vi "_r2dio_8in_8out_canopen_master.vi"() -> ()   [LabVIEW 2011]
uses:
  CANopen_VI/stop_can_master.vi
panel:
  out "ret transmit_can_pdo":i16
  out "datasize":u32
  out "Manufacturer software ver":string
  out "ret read_device_object_sdo 3":i16
  out "datasize":u32
  out "Manufacturer hardware ver":string
  out "ret read_device_object_sdo 2":i16
  out "datasize":u32
  out "Manufacturer dev name":string
  out "ret read_device_object_sdo 1":i16
  out "ret write_node_object_dictionary":i16
  in  "7":bool
  in  "6":bool
  in  "5":bool
  in  "4":bool
  in  "3":bool
  in  "2":bool
  in  "1":bool
  in  "0":bool
  out "ret write_pdo_mapping 6":i16
  out "ret write_pdo_mapping 5":i16
  out "ret write_pdo_mapping 4":i16
  out "ret add_node_object_dictionary 6200":i16
  out "7":bool
  out "6":bool
  out "5":bool
  out "4":bool
  out "3":bool
  out "2":bool
  out "1":bool
  out "0":bool
  out "7":bool
  out "6":bool
  out "5":bool
  out "4":bool
  out "3":bool
  out "2":bool
  out "1":bool
  out "0":bool
  out "uns8":u8
  out "upd":u8
  out "ret read_node_object_dictionary":i16
  in  "stop monitor":bool
  out "ret write_master_hbt":i16
  out "ret stop_can_master":i16
  out "ret write_pdo_mapping 3":i16
  out "ret write_pdo_mapping 2":i16
  out "ret write_pdo_mapping 1":i16
  out "ret add_node_object_dictionary 6000":i16
  out "ret write_device_object_sdo":i16
  in  "slave node":u8
  in  "baudrate":T1(ring)
  in  "net":u8
  # "Inputs"
  # "Outputs"
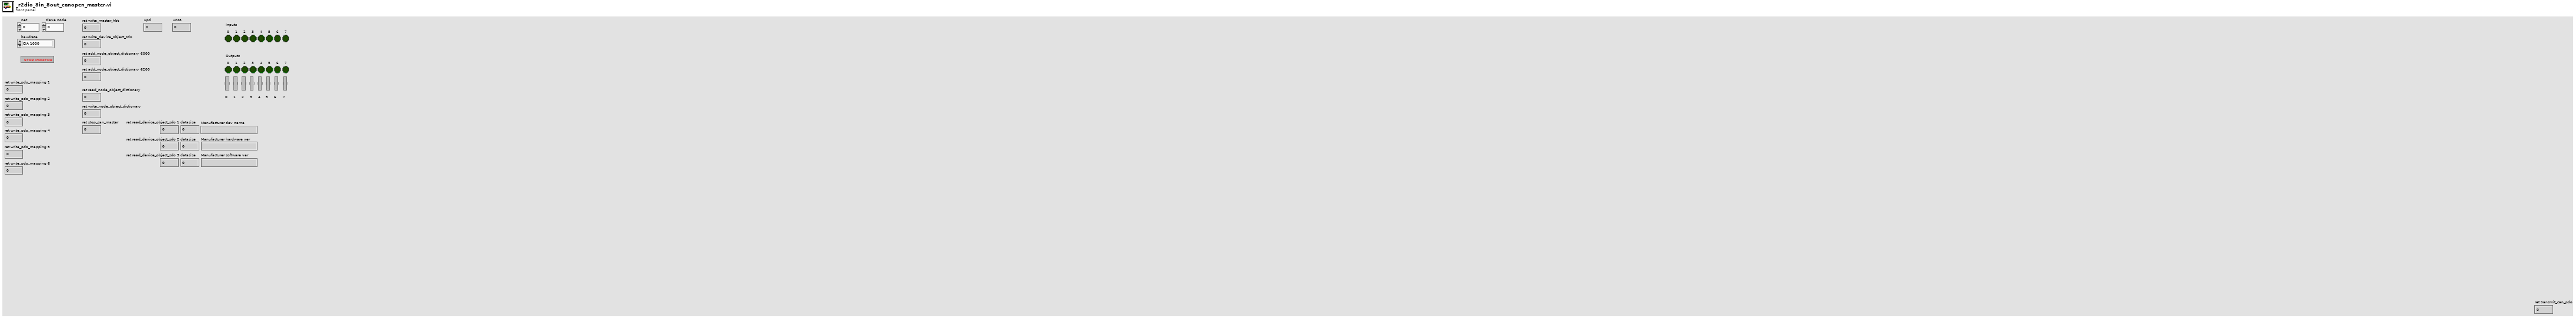
[diagram p1: front panel]
types:
  T1 = enum8{"CIA 1000", "CIA 800", "CIA 500", "CIA 250", "CIA 125", "CIA 100", "CIA 50", "CIA 20", "CIA 10", "CIA AUTO"}
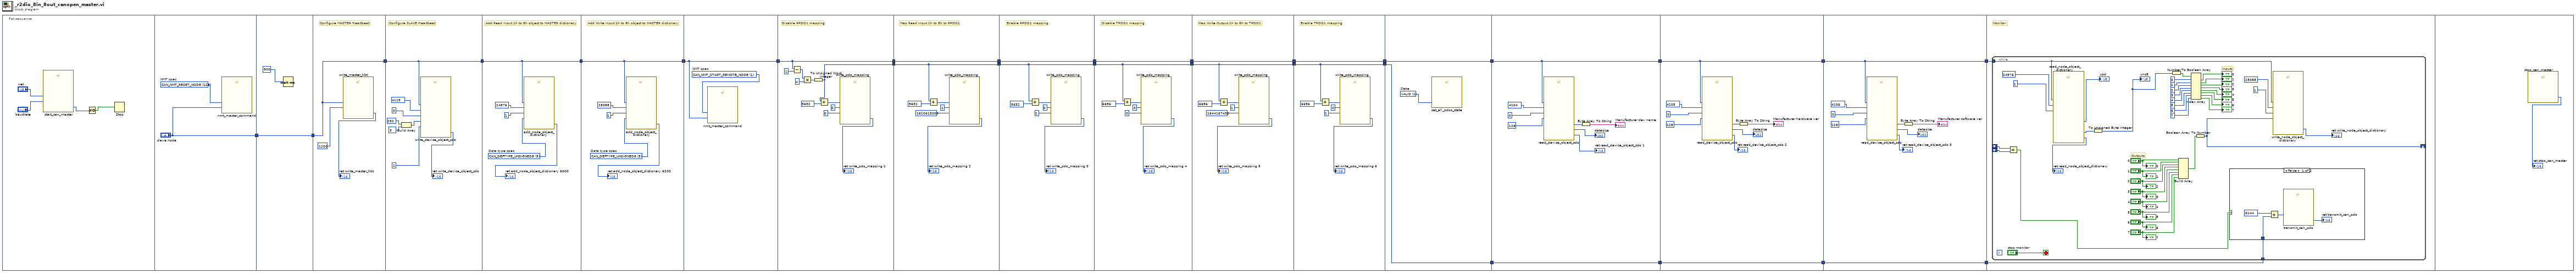
[diagram p0: block diagram]
diagram:
  n1 = flat-sequence {
    tunnel: ["slave node"] -> w25
    tunnel: w25 -> [w35]
    tunnel: [w35] -> w24
    tunnel: w24 -> [w37]
    tunnel: [w37] -> w27
    tunnel: w27 -> [w44]
    tunnel: [w44] -> w26
    tunnel: w26 -> [w47]
    tunnel: [w47] -> w20
    tunnel: w20 -> [w52]
    tunnel: [w52] -> w19
    tunnel: [w57] -> w21
    tunnel: w19 -> [w57]
    tunnel: [w62] -> w22
    tunnel: w21 -> [w62]
    tunnel: [w59] -> w10
    tunnel: [w73] -> w23
    tunnel: w22 -> [w73]
    tunnel: w10 -> [w70]
    tunnel: [w70] -> w9
    tunnel: [w80] -> w18
    tunnel: w23 -> [w80]
    tunnel: w9 -> [w77]
    tunnel: [w77] -> w8
    tunnel: w18 -> [w90]
    tunnel: [w90] -> w17
    tunnel: w8 -> [w84]
    tunnel: [w84] -> w7
    tunnel: w17 -> [w97]
    tunnel: [w97] -> w16
    tunnel: w7 -> [w91]
    tunnel: [w91] -> w6
    tunnel: w16 -> [w104]
    tunnel: [w104] -> w15
    tunnel: w6 -> [w98]
    tunnel: [w98] -> w1
    tunnel: [w106] -> w14
    tunnel: w15 -> [w106]
    tunnel: [w105] -> w2
    tunnel: w1 -> [w105]
    tunnel: w14 -> [w116]
    tunnel: [w116] -> w13
    tunnel: [w108] -> w3
    tunnel: w2 -> [w108]
    tunnel: w13 -> [w118]
    tunnel: [w118] -> w12
    tunnel: [w117] -> w4
    tunnel: w3 -> [w117]
    tunnel: w12 -> [w127]
    tunnel: [w127] -> w11
    tunnel: [w126] -> w5
    tunnel: w4 -> [w126]
    tunnel: w11 -> [w136]
    tunnel: w5 -> [w135]
    frame #0 {
      n2 = call "start_can_master.vi"("br"="baudrate", "net"="net") -> ("return"=w31:i16)  [unwired: 9 in]
      n3 = Not Equal To 0?(x=w31) -> (x != 0?=w30:bool)
      n4 = Stop(stop? (T)=w30) -> ()
    }
    frame #1 {
      w33 = u8 129 items=["CAN_NMT_CS_DUMMY"=0, "CAN_NMT_START_REMOTE_NODE"=1, "CAN_NMT_STOP_REMOTE_NODE"=2, "CAN_NMT_ENTER_PRE_OPERATIONAL"=128, "CAN_NMT_RESET_NODE"=129, "CAN_NMT_RESET_COMMUNICATION"=130]  # NMT spec
      n5 = call "nmt_master_command.vi"("node"="slave node", "cs"=w33) -> ()  [unwired: 10 in]
    }
    frame #2 {
      n6 = Wait (ms)(milliseconds to wait=u32 500) -> ()  [unwired: 1 out]
    }
    frame #3 {
      # "Configure MASTER Heartbeat"
      n7 = call "write_master_hbt.vi"("hbt"=u16 1200, "node"=w37) -> ("return"=→"ret write_master_hbt":i16)  [unwired: 9 in]
    }
    frame #4 {
      # "Configure SLAVE Heartbeat"
      n8 = Build Array(u8 232, u8 3) -> (w40:u8[])
      n9 = call "write_device_object_sdo.vi"("node"=w44, "index"=u16 4119, "subind"=u8 0, "data"=w40, "datasize"=u32 2) -> ("return"=→"ret write_device_object_sdo":i16)  [unwired: 10 in]
    }
    frame #5 {
      w49 = u16 5 items=["CAN_DEFTYPE_BOOLEAN"=1, "CAN_DEFTYPE_INTEGER8"=2, "CAN_DEFTYPE_INTEGER16"=3, "CAN_DEFTYPE_INTEGER32"=4, "CAN_DEFTYPE_UNSIGNED8"=5, "CAN_DEFTYPE_UNSIGNED16"=6, "CAN_DEFTYPE_UNSIGNED32"=7, "CAN_DEFTYPE_REAL32"=8, "CAN_DEFTYPE_VISIBLE_STRING"=9, "CAN_DEFTYPE_OCTET_STRING"=10, "CAN_DEFTYPE_UNICODE_STRING"=11, "CAN_DEFTYPE_TIME_OF_DAY"=12, "CAN_DEFTYPE_TIME_DIFFERENCE"=13, "CAN_DEFTYPE_DOMAIN"=15, "CAN_DEFTYPE_INTEGER24"=16, "CAN_DEFTYPE_REAL64"=17, "CAN_DEFTYPE_INTEGER40"=18, "CAN_DEFTYPE_INTEGER48"=19, "CAN_DEFTYPE_INTEGER56"=20, "CAN_DEFTYPE_INTEGER64"=21, "CAN_DEFTYPE_UNSIGNED24"=22, "CAN_DEFTYPE_UNSIGNED40"=24, "CAN_DEFTYPE_UNSIGNED48"=25, "CAN_DEFTYPE_UNSIGNED56"=26, "CAN_DEFTYPE_UNSIGNED64"=27]  # Data type spec
      # "Add Read Input 1h to 8h object to MASTER dictionary"
      n10 = call "add_node_object_dictionary.vi"("type"=w49, "subind"=u8 1, "index"=u16 24576, "node"=w47) -> ("return"=→"ret add_node_object_dictionary 6000":i16)  [unwired: 7 in]
    }
    frame #6 {
      w54 = u16 5 items=["CAN_DEFTYPE_BOOLEAN"=1, "CAN_DEFTYPE_INTEGER8"=2, "CAN_DEFTYPE_INTEGER16"=3, "CAN_DEFTYPE_INTEGER32"=4, "CAN_DEFTYPE_UNSIGNED8"=5, "CAN_DEFTYPE_UNSIGNED16"=6, "CAN_DEFTYPE_UNSIGNED32"=7, "CAN_DEFTYPE_REAL32"=8, "CAN_DEFTYPE_VISIBLE_STRING"=9, "CAN_DEFTYPE_OCTET_STRING"=10, "CAN_DEFTYPE_UNICODE_STRING"=11, "CAN_DEFTYPE_TIME_OF_DAY"=12, "CAN_DEFTYPE_TIME_DIFFERENCE"=13, "CAN_DEFTYPE_DOMAIN"=15, "CAN_DEFTYPE_INTEGER24"=16, "CAN_DEFTYPE_REAL64"=17, "CAN_DEFTYPE_INTEGER40"=18, "CAN_DEFTYPE_INTEGER48"=19, "CAN_DEFTYPE_INTEGER56"=20, "CAN_DEFTYPE_INTEGER64"=21, "CAN_DEFTYPE_UNSIGNED24"=22, "CAN_DEFTYPE_UNSIGNED40"=24, "CAN_DEFTYPE_UNSIGNED48"=25, "CAN_DEFTYPE_UNSIGNED56"=26, "CAN_DEFTYPE_UNSIGNED64"=27]  # Data type spec
      # "Add Write Input 1h to 8h object to MASTER dictionary"
      n11 = call "add_node_object_dictionary.vi"("type"=w54, "subind"=u8 1, "index"=u16 25088, "node"=w52) -> ("return"=→"ret add_node_object_dictionary 6200":i16)  [unwired: 7 in]
    }
    frame #7 {
      w58 = u8 1 items=["CAN_NMT_CS_DUMMY"=0, "CAN_NMT_START_REMOTE_NODE"=1, "CAN_NMT_STOP_REMOTE_NODE"=2, "CAN_NMT_ENTER_PRE_OPERATIONAL"=128, "CAN_NMT_RESET_NODE"=129, "CAN_NMT_RESET_COMMUNICATION"=130]  # NMT spec
      n12 = call "nmt_master_command.vi"("node"=w57, "cs"=w58) -> ()  [unwired: 10 in]
    }
    frame #8 {
      # "Disable RPDO1 mapping"
      n13 = Subtract(x=w62, y=u8 1) -> (x-y=w64:u8)
      n14 = Multiply(x=w64, y=u8 4) -> (x*y=w63:u8)
      n15 = To Unsigned Word Integer(number=w63) -> (unsigned 16bit integer=w59:u16)
      n16 = Add(x=w59, y=u16 5632) -> (x+y=w61:u16)
      n17 = call "write_pdo_mapping.vi"("data"=u32 0, "subind"=u8 0, "index"=w61) -> ("return"=→"ret write_pdo_mapping 1":i16)  [unwired: 8 in]
    }
    frame #9 {
      # "Map Read Input 1h to 8h to RPDO1"
      n18 = Add(x=w70, y=u16 5632) -> (x+y=w72:u16)
      n19 = call "write_pdo_mapping.vi"("data"=u32 1610613000, "subind"=u8 1, "index"=w72) -> ("return"=→"ret write_pdo_mapping 2":i16)  [unwired: 8 in]
    }
    frame #10 {
      # "Enable RPDO1 mapping"
      n20 = Add(x=w77, y=u16 5632) -> (x+y=w79:u16)
      n21 = call "write_pdo_mapping.vi"("data"=u32 1, "subind"=u8 0, "index"=w79) -> ("return"=→"ret write_pdo_mapping 3":i16)  [unwired: 8 in]
    }
    frame #11 {
      # "Disable TPDO1 mapping"
      n22 = Add(x=w84, y=u16 6656) -> (x+y=w86:u16)
      n23 = call "write_pdo_mapping.vi"("data"=u32 0, "subind"=u8 0, "index"=w86) -> ("return"=→"ret write_pdo_mapping 4":i16)  [unwired: 8 in]
    }
    frame #12 {
      # "Map Write Output 1h to 8h to TPDO1"
      n24 = Add(x=w91, y=u16 6656) -> (x+y=w93:u16)
      n25 = call "write_pdo_mapping.vi"("data"=u32 1644167432, "subind"=u8 1, "index"=w93) -> ("return"=→"ret write_pdo_mapping 5":i16)  [unwired: 8 in]
    }
    frame #13 {
      # "Enable TPDO1 mapping"
      n26 = Add(x=w98, y=u16 6656) -> (x+y=w100:u16)
      n27 = call "write_pdo_mapping.vi"("data"=u32 1, "subind"=u8 0, "index"=w100) -> ("return"=→"ret write_pdo_mapping 6":i16)  [unwired: 8 in]
    }
    frame #14 {
      w107 = u8 1 items=["NOT_VALID", "VALID"]  # State
      n28 = call "set_all_pdos_state.vi"("state"=w107) -> ()  [unwired: 11 in]
    }
    frame #15 {
      n29 = call "read_device_object_sdo.vi"("node"=w116, "index"=u16 4104, "subind"=u8 0, "datasize"=u32 128) -> ("return"=→"ret read_device_object_sdo 1":i16, "data"=w111:u8[], "datasize"=→"datasize":u32)  [unwired: 9 in]
      n30 = Byte Array To String(unsigned byte array=w111) -> (string=→"Manufacturer dev name":string)
    }
    frame #16 {
      n31 = call "read_device_object_sdo.vi"("node"=w118, "index"=u16 4105, "subind"=u8 0, "datasize"=u32 128) -> ("return"=→"ret read_device_object_sdo 2":i16, "data"=w121:u8[], "datasize"=→"datasize":u32)  [unwired: 9 in]
      n32 = Byte Array To String(unsigned byte array=w121) -> (string=→"Manufacturer hardware ver":string)
    }
    frame #17 {
      n33 = call "read_device_object_sdo.vi"("node"=w127, "index"=u16 4106, "subind"=u8 0, "datasize"=u32 128) -> ("return"=→"ret read_device_object_sdo 3":i16, "data"=w130:u8[], "datasize"=→"datasize":u32)  [unwired: 9 in]
      n34 = Byte Array To String(unsigned byte array=w130) -> (string=→"Manufacturer software ver":string)
    }
    frame #18 {
      # "Monitor"
      n35 = while {
        tunnel: w136 -> [w156]
        shift-right: [w141] -> _
        shift-left: _ -> [w140]
        shift-left: _ -> [w139]
        tunnel: w135 -> [w137]
        stop <- "stop monitor" stop-if-true
        # "Outputs"
        # "Inputs"
        n36 = Equal?(x=w140, y=w139) -> (x = y?=w138:bool)
        n37 = call "read_node_object_dictionary.vi"("node"=w156, "index"=u16 24576, "subind"=u8 1) -> ("return"=→"ret read_node_object_dictionary":i16, "upd"=→"upd":u8, "num"=w144:u64)  [unwired: 10 in]
        n38 = To Unsigned Byte Integer(number=w144) -> (unsigned 8bit integer=w143:u8)
        "uns8" <- w143
        n39 = Number To Boolean Array(number=w143) -> (Boolean array=w165:bool[])
        n40 = Build Array("0", "1", "2", "3", "4", "5", "6", "7") -> (w145:bool[])
        n41 = Index Array(array=w165, index #1=0, index #2=1, index #3=2, index #4=3, index #5=4, index #6=5, index #7=6, index #8=7) -> (element #1=→"0":bool, element #2=→"1":bool, element #3=→"2":bool, element #4=→"3":bool, element #5=→"4":bool, element #6=→"5":bool, element #7=→"6":bool, element #8=→"7":bool)
        n42 = Boolean Array To Number(Boolean array=w145) -> (number=w141:u64)
        n43 = case shown="False" w138 {
          tunnel: w137 -> [w180 _]
          frame False {
            n44 = Add(x=u16 6144, y=w180) -> (x+y=w181:u16)
            n45 = call "transmit_can_pdo.vi"("index"=w181) -> ("return"=→"ret transmit_can_pdo":i16)  [unwired: 10 in]
          }
          frame True {
          }
        }
        n46 = call "write_node_object_dictionary.vi"("num"=w141, "subind"=u8 1, "index"=u16 25088, "node"=w156) -> ("return"=→"ret write_node_object_dictionary":i16)  [unwired: 6 in, 1 out]
        "0" <- "0"
        "1" <- "1"
        "2" <- "2"
        "3" <- "3"
        "4" <- "4"
        "5" <- "5"
        "6" <- "6"
        "7" <- "7"
      }
    }
    frame #19 {
      n47 = call "stop_can_master"() -> ("return"=→"ret stop_can_master":i16)  [unwired: 11 in]
    }
  }
